vi "Insert Run.vi"(6 "Reinsert?":bool, 8 "error in (no error)":errorcluster, 9 "Repetitions":u32=1, 10 "Run Instance":refnum<class "Run Instance.lvclass">, 11 "Schedule in":refnum<class "Schedule.lvclass">) -> (0 "error out":errorcluster, 2 "Index":i32, 3 "Schedule out":refnum<class "Schedule.lvclass">)   [LabVIEW 2020, in "Run Utilities.lvlib" / "Schedule.lvclass"]
doc: "Vi for inserting single Run Instance into the schedule. It either increseas the number of repetitions on the existing entry or appends it to the array as a new entry. If the Reinsert is True, it adds the script at first position, otherwise it adds it at the end."
uses:
  Schedule.lvclass
  Run Instance/Run Instance.lvclass
  Schedule.lvclass/Schedule.ctl
  Cell/Schedule Cell.lvclass
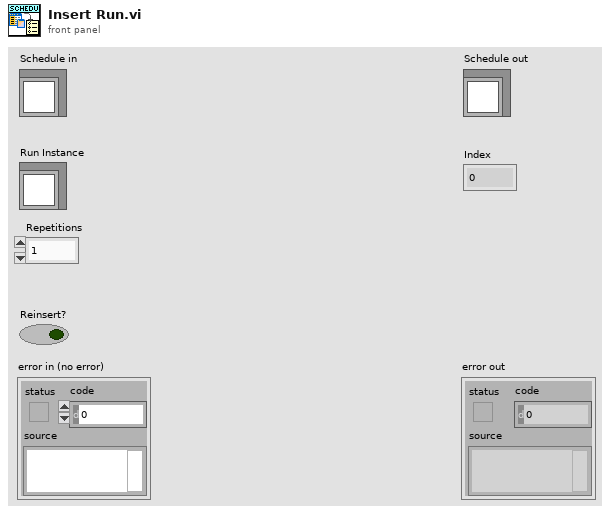
[diagram p1: front panel]
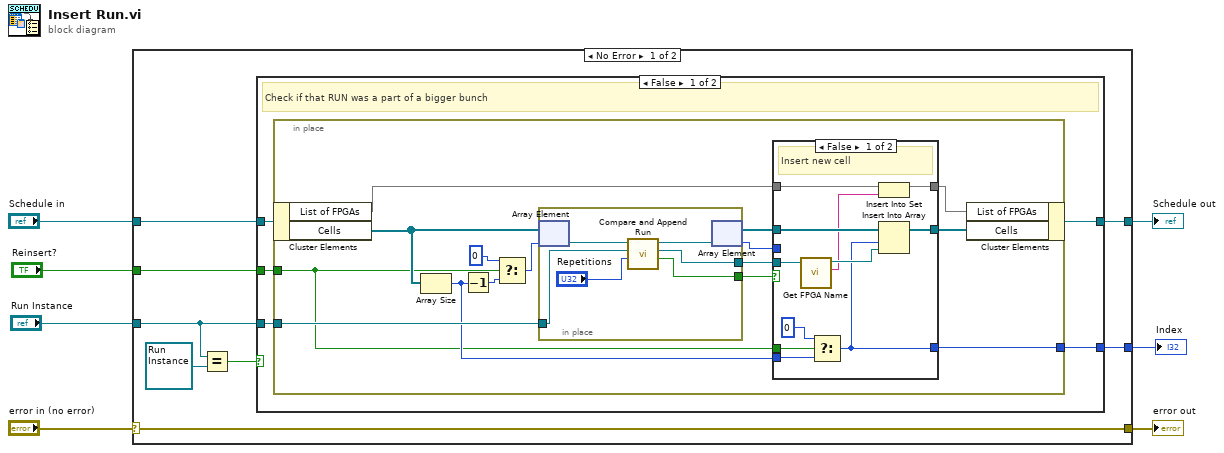
[diagram p0: block diagram]
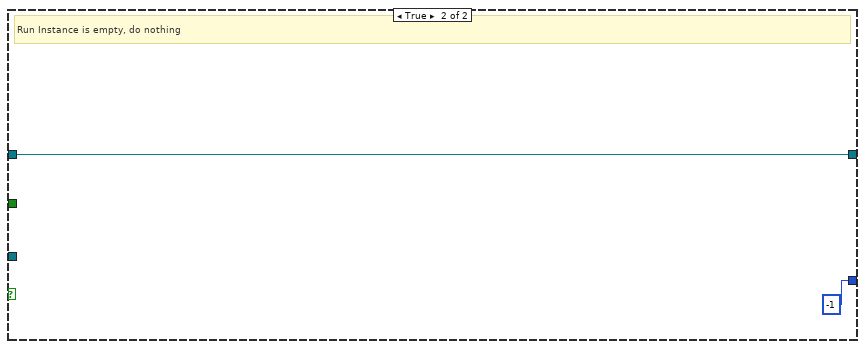
[diagram p3: hidden frame]
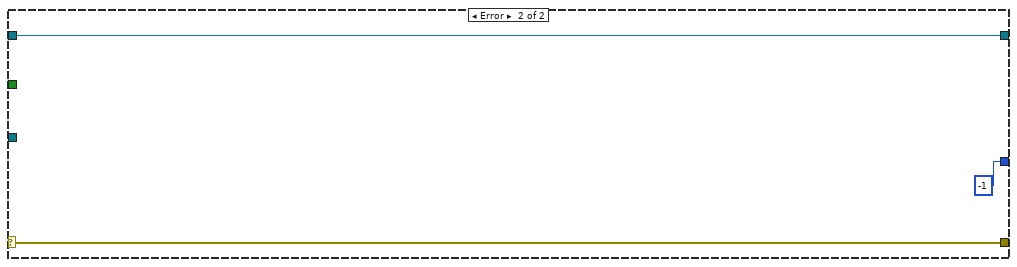
[diagram p4: hidden frame]
diagram:
  n1 = case shown="No Error" "error in (no error)" {
    selector: "error in (no error)" -> [w14 w60]
    tunnel: [w14 w60] -> w6
    tunnel: [w13 w59] -> w4
    tunnel: "Schedule in" -> [w15 w59]
    tunnel: "Run Instance" -> [w12 _]
    tunnel: "Reinsert?" -> [w9 _]
    tunnel: [w8 -1 ("t")] -> w1
    frame No Error {
      n2 = Equal?(x=w12, y=refnum<class "Run Instance.lvclass"> refnum ("Run Instance")) -> (x = y?=w10:bool)
      n3 = case shown="False" w10 {
        tunnel: w15 -> [w17 w57]
        tunnel: [w16 w57] -> w13
        tunnel: w12 -> [w20 _]
        tunnel: w9 -> [w19 _]
        tunnel: [w18 -1 ("t")] -> w8
        frame False {
          # "Check if that RUN was a part of a bigger bunch"
          n4 = in-place {
            in-place-border: w20 -> [w35]
            in-place-border: w19 -> [w21]
            in-place-border: [w27] -> w18
            n5 = in-place-cluster #1(w17) -> ("List of FPGAs"=w23:set{string}, "Cells"=w25:refnum<class "Schedule Cell.lvclass">[])
            n6 = Array Size(array=w25) -> (size(s)=w28:i32)
            n7 = Decrement(x=w28) -> (x-1=w34:i32)
            n8 = Select(t=0, s=w21, f=w34) -> (s? t:f=w32:i32)
            n9 = in-place {
              in-place-border: w35 -> [w53]
              in-place-border: [w52] -> w30
              in-place-border: [w51] -> w29
              n10 = in-place-array #2(w25, w32) -> (w55:refnum<class "Schedule Cell.lvclass">)
              n11 = call-dynamic "Compare and Append Run.vi"("Repetitions"="Repetitions", "Run"=w53, "Schedule Cell in"=w55) -> ("Cell Updated"=w51:bool, "new Schedule Cell out"=w52:refnum<class "Schedule Cell.lvclass">, "Schedule Cell out"=w54:refnum<class "Schedule Cell.lvclass">)  [unwired: 5 in, 1 out]
              n12 = in-place-array #2(w54) -> (w31:refnum<class "Schedule Cell.lvclass">[], w26:i32)
            }
            n13 = case shown="False" w29 {
              tunnel: w31 -> [w45 w49]
              tunnel: w30 -> [w37 _]
              tunnel: [w44 w49] -> w24
              tunnel: w21 -> [w43 _]
              tunnel: w28 -> [w42 _]
              tunnel: [w40 w48] -> w27
              tunnel: w26 -> [_ w48]
              tunnel: w23 -> [w39 w47]
              tunnel: [w38 w47] -> w22
              frame False {
                # "Insert new cell"
                n14 = call-dynamic "Get FPGA Name.vi"("Schedule Cell in"=w37) -> ("FPGA Name"=w36:string, "Schedule Cell out"=w46:refnum<class "Schedule Cell.lvclass">)  [unwired: 8 in, 1 out]
                n15 = Select(t=0, s=w43, f=w42) -> (s? t:f=w40:i32)
                n16 = Insert Into Set(10:w36, 11:w39) -> (3:w38:set{string})  [unwired: 1 out]
                n17 = Insert Into Array(array=w45, index=w40, new element=w46) -> (w44:refnum<class "Schedule Cell.lvclass">[])
              }
              frame True {
                # "Updated cell"
              }
            }
            n18 = in-place-cluster #1("List of FPGAs"=w22, "Cells"=w24) -> (w16:refnum<class "Schedule.lvclass">)
          }
        }
        frame True {
          # "Run Instance is empty, do nothing"
        }
      }
    }
    frame Error {
    }
  }
  "error out" <- w6
  "Schedule out" <- w4
  "Index" <- w1
